vi "LSCI332 SetSetpoint.vi"(0 "VISA Rsrc":refnum<visa-resource-name>="GPIB0::12::INSTR", 5 "Boucle(1)":u32(ring) caption="Boucle" items=["Boucle 1", "Boucle 2"], 7 "SetPoint":dbl, 11 "error in (no error)":errorcluster) -> (15 "error out":errorcluster)   [LabVIEW 2019]
doc: "Ce VI écrit les paramètres limites de contrôle dans le contrôleur."
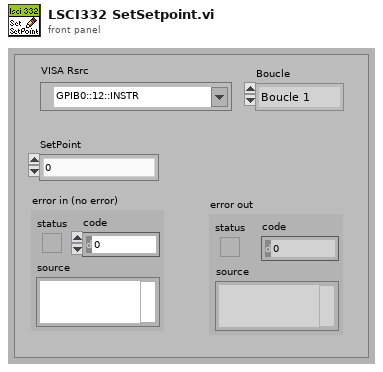
[diagram p1: front panel]
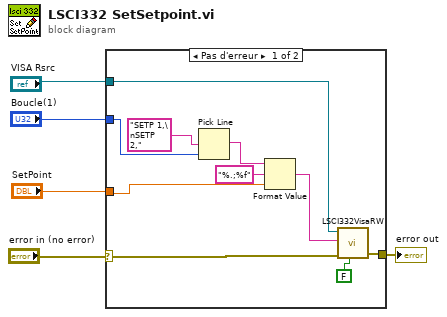
[diagram p0: block diagram]
diagram:
  n1 = case shown="Pas d'erreur" "error in (no error)" {
    selector: "error in (no error)" -> [w13 w16]
    tunnel: "VISA Rsrc" -> [w15 _]
    tunnel: "Boucle(1)" -> [w10 _]
    tunnel: [w14 w16] -> w3
    tunnel: "SetPoint" -> [w8 _]
    frame No Error {
      n2 = Pick Line(multi-line string="SETP 1,\nSETP 2,", line index=w10) -> (output string=w9:string)  [unwired: 1 in]
      n3 = Format Value(string ("")=w9, format string="%.;%f", value (0)=w8) -> (output string=w6:string)
      n4 = call <userlib>:"LSCI332VisaRW.vi"("Lecture?(T)"=FALSE, "error in (no error)"=w13, "ChaineCom"=w6, "VISA Rsrc"=w15) -> ("error out"=w14:errorcluster)  [unwired: 3 in, 3 out]
    }
    frame Error {
    }
  }
  "error out" <- w3
